vi "Inficon Basic Tester.vi"(8 "Error In":errorcluster, 11 "Remote IP Address":string="192.168.1.32") -> (0 "Error Out":errorcluster, 3 "Inficon Data Output":T1)   [LabVIEW 2020]
uses:
  Type Definitions/Inficon Data.ctl
  <vilib>/NI/Modbus Library/API/Wrapper/Create TCP Master.vi
  <vilib>/NI/Modbus Library/API/Master/Modbus Master.lvclass
  <vilib>/NI/Modbus Library/API/Wrapper/API Main.lvlib
panel:
  # "NG Inficon: 192.168.1.32\nLP Inficon: 192.168.1.33"
  # "Natural Gas"
  # "Propane"
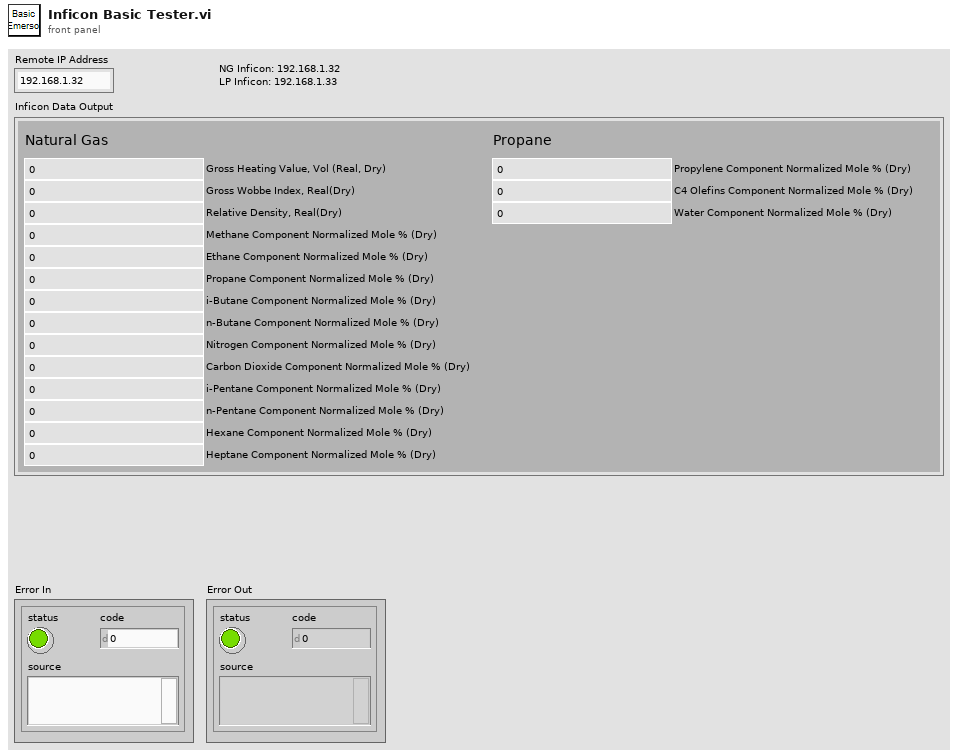
[diagram p1: front panel]
types:
  T1 = typedef "Inficon Data.ctl" = cluster{"Gross Heating Value, Vol (Real, Dry)":dbl, "Nitrogen Component Normalized Mole % (Dry)":dbl, "Methane Component Normalized Mole % (Dry)":dbl, "Carbon Dioxide Component Normalized Mole % (Dry)":dbl, "Ethane Component Normalized Mole % (Dry)":dbl, "Propane Component Normalized Mole % (Dry)":dbl, "i-Pentane Component Normalized Mole % (Dry)":dbl, "i-Butane Component Normalized Mole % (Dry)":dbl, "n-Butane Component Normalized Mole % (Dry)":dbl, "n-Pentane Component Normalized Mole % (Dry)":dbl, "Hexane Component Normalized Mole % (Dry)":dbl, "Heptane Component Normalized Mole % (Dry)":dbl, "Gross Wobbe Index, Real(Dry)":dbl, "Relative Density, Real(Dry)":dbl, "Propylene Component Normalized Mole % (Dry)":dbl, "C4 Olefins Component Normalized Mole % (Dry)":dbl, "Water Component Normalized Mole % (Dry)":dbl}
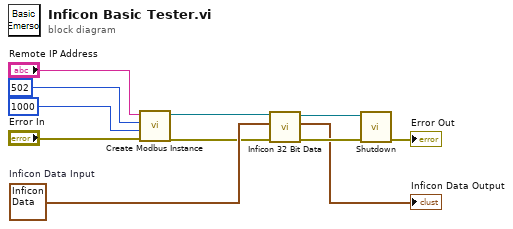
[diagram p0: block diagram]
diagram:
  w3 = T1 {"Gross Heating Value, Vol (Real, Dry)"=0.0, "Nitrogen Component Normalized Mole % (Dry)"=0.0, "Methane Component Normalized Mole % (Dry)"=0.0, "Carbon Dioxide Component Normalized Mole % (Dry)"=0.0, "Ethane Component Normalized Mole % (Dry)"=0.0, "Propane Component Normalized Mole % (Dry)"=0.0, "i-Pentane Component Normalized Mole % (Dry)"=0.0, "i-Butane Component Normalized Mole % (Dry)"=0.0, "n-Butane Component Normalized Mole % (Dry)"=0.0, "n-Pentane Component Normalized Mole % (Dry)"=0.0, "Hexane Component Normalized Mole % (Dry)"=0.0, "Heptane Component Normalized Mole % (Dry)"=0.0, "Gross Wobbe Index, Real(Dry)"=0.0, "Relative Density, Real(Dry)"=0.0, "Propylene Component Normalized Mole % (Dry)"=0.0, "C4 Olefins Component Normalized Mole % (Dry)"=0.0, "Water Component Normalized Mole % (Dry)"=0.0}  # Inficon Data Input
  n1 = call-poly <vilib>:"Create Modbus Instance.vi"("error in"="Error In", "connect timeout ms"=1000, "port (502)"=u16 502, "address"="Remote IP Address") -> ("error out"=w2:errorcluster, "TCP master instance"=w4:refnum<class "Modbus Master.lvclass">)  [unwired: 6 in]
  n2 = call "Inficon 32 Bit Data.vi"("Error In"=w2, "Inficon Data Input"=w3, "Modbus master in"=w4) -> ("Error Out"=w9:errorcluster, "Inficon Data Output"=→"Inficon Data Output":T1, "Modbus master out"=w8:refnum<class "Modbus Master.lvclass">)  [unwired: 5 in, 1 out]
  n3 = call-dynamic "Shutdown.vi"("error in"=w9, "Modbus master in"=w8) -> ("error out"=→"Error Out":errorcluster)  [unwired: 9 in]
